vi "initialise.vi"(8 "error in (no error)":errorcluster, 11 "ImageAssemblerRK110612 in":refnum<class "ImageAssemblerRK110612Spiral.lvclass">) -> (0 "error out":errorcluster, 3 "ImageAssemblerRK110612 out":refnum<class "ImageAssemblerRK110612Spiral.lvclass">)   [LabVIEW 2010, in "ImageAssemblerRK110612Spiral.lvclass"]
doc: "The dynamic dispatch-version of this VI initalises the plug-in object by allocating and initalising any dynamic resources need."
uses:
  ImageAssemblerRK110612Spiral.lvclass
  ImageAssemblerDL090211Scaffold/ImageAssemblerDL090211Scaffold/ImageAssemblerDL090211Scaffold.lvclass
  ImageAssemblerRK110612Spiral.lvclass/ImageAssemblerRK110612Spiral.ctl
  DAQ/GenericDAQ/GenericDAQ/GenericDAQ.lvclass
  common/classes/GenericComponent/GenericComponent/GenericComponent.lvclass
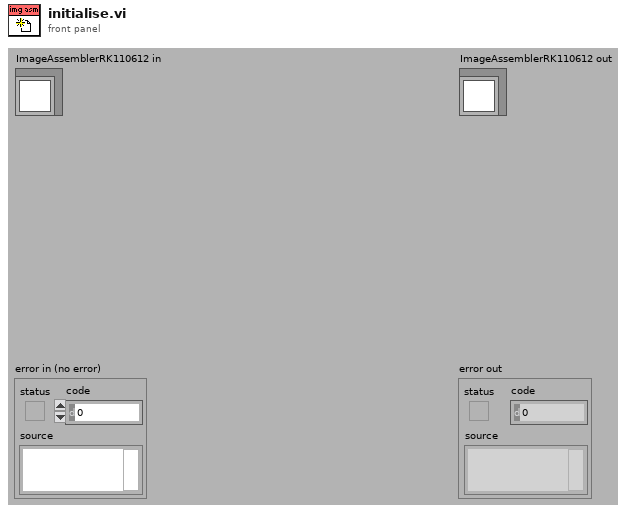
[diagram p1: front panel]
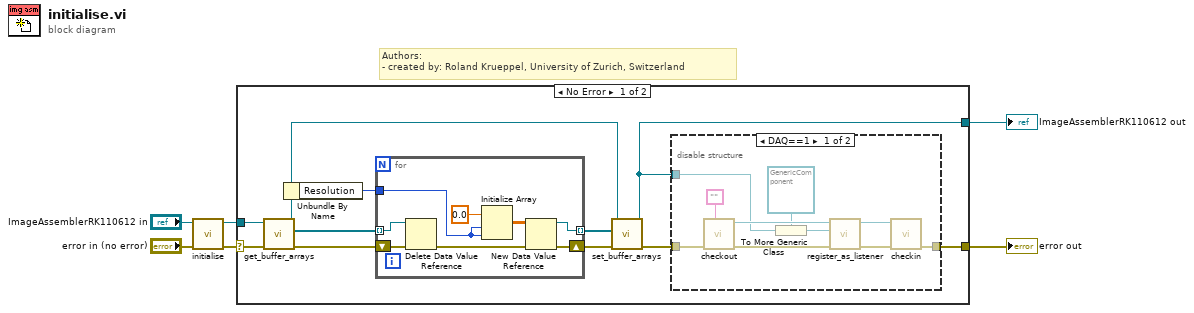
[diagram p0: block diagram]
diagram:
  # "Authors: \n- created by: Roland Krueppel, University of Zurich, Switzerland"
  n1 = call-parent "initialise.vi"("error in (no error)"="error in (no error)", "GenericPlugin in"="ImageAssemblerRK110612 in") -> ("error out"=w4:errorcluster, "GenericPlugin out"=w2:refnum<class "ImageAssemblerRK110612Spiral.lvclass">)  [unwired: 8 in]
  n2 = case shown="No Error" w4 {
    selector: w4 -> [w16 w38]
    tunnel: [w17 w38] -> w3
    tunnel: w2 -> [w14 w37]
    tunnel: [w11 w37] -> w1
    frame No Error {
      n3 = call-dynamic "get_buffer_arrays.vi"("error in (no error)"=w16, "ImageAssemblerRK110612Spiral in"=w14) -> ("error out"=w15:errorcluster, "Buffer arrays"=w10:refnum<data-value>[], "ImageAssemblerRK110612Spiral out"=w9:refnum<class "ImageAssemblerRK110612Spiral.lvclass">)  [unwired: 7 in]
      n4 = Unbundle By Name(w9) -> ("Resolution"=w8:i32)
      n5 = for {
        tunnel: w8 -> [w22]
        tunnel: w10 -> [w19] mode=indexing
        tunnel: [w18] -> w7 mode=indexing
        shift-right: [w20] -> w13
        shift-left: w15 -> [w21]
        n6 = Delete Data Value Reference(data value reference=w19, error in=w21) -> (error out=w23:errorcluster)  [unwired: 1 out]
        n7 = Initialize Array(sgl 0.0 ("element"), w22, w22) -> (w24:sgl[][])
        n8 = New Data Value Reference(data value=w24, error in=w23) -> (data value reference=w18:refnum<data-value>, error out=w20:errorcluster)
      }
      n9 = call-dynamic "set_buffer_arrays.vi"("error in (no error)"=w13, "Buffer arrays"=w7, "ImageAssemblerRK110612Spiral in"=w9) -> ("error out"=w12:errorcluster, "ImageAssemblerRK110612Spiral out"=w11:refnum<class "ImageAssemblerRK110612Spiral.lvclass">)  [unwired: 7 in]
      n10 = disable-structure shown="DAQ==1" {
        disable-tunnel: w11 -> [w30 _]
        disable-tunnel: w12 -> [w35 w36]
        disable-tunnel: [w26 w36] -> w17
        frame condition #0 {
          n11 = call "checkout.vi"("locked by?"="", "error in (no error)"=w35) -> ("error out"=w33:errorcluster, "GenericDAQ out"=w32:refnum<class "GenericDAQ.lvclass">)  [unwired: 8 in]
          n12 = To More Generic Class(target class=refnum<class "GenericComponent.lvclass"> refnum ("GenericComponent.lvclass"), reference=w30) -> (generic class reference=w31:refnum<class "GenericComponent.lvclass">)
          n13 = call-dynamic "register_as_listener.vi"("error in (no error)"=w33, "GenericComponent.lvclass"=w31, "GenericDAQ in"=w32) -> ("error out"=w27:errorcluster, "GenericDAQ out"=w28:refnum<class "GenericDAQ.lvclass">)  [unwired: 7 in]
          n14 = call "checkin.vi"("error in (no error)"=w27, "GenericDAQ in"=w28) -> ("error out"=w26:errorcluster)  [unwired: 8 in, 1 out]
        }
        frame condition #1 (active) {
        }
      }
    }
    frame Error {
    }
  }
  "error out" <- w3
  "ImageAssemblerRK110612 out" <- w1
